vi "HandleRollerPneumatic.vi"(8 "error in (no error)":errorcluster, 10 "InitState":T1=enum."Middle", 11 "Toggle?":bool) -> (0 "error out":errorcluster, 2 "State":T1, 3 "Enqueue?":bool)   [LabVIEW 2013]
uses:
  Robot_Framework_2014/DoubleSolenoidAction.ctl
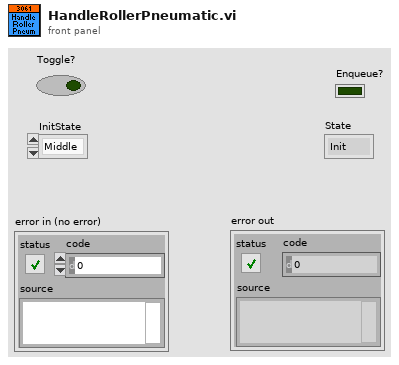
[diagram p1: front panel]
types:
  T1 = typedef "DoubleSolenoidAction.ctl" = enum16{"Init", "Middle", "In", "Out"}
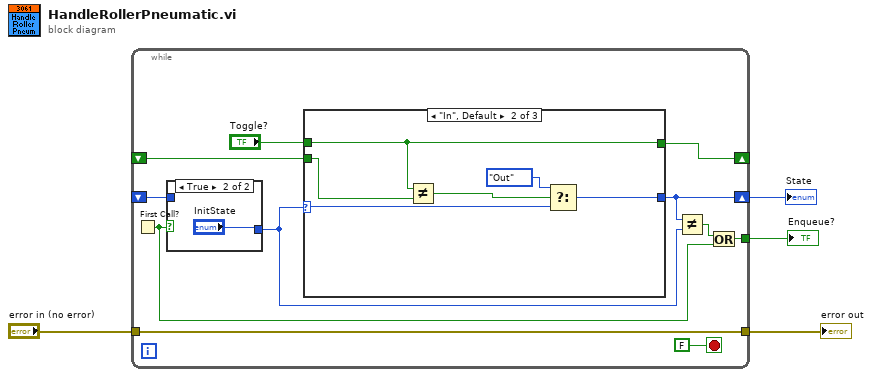
[diagram p0: block diagram]
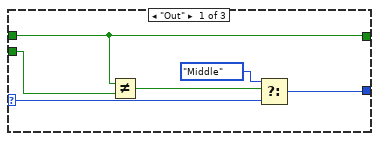
[diagram p3: hidden frame]
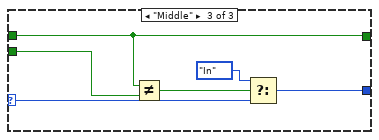
[diagram p4: hidden frame]
diagram:
  n1 = while {
    shift-right: [w9] -> w4
    shift-left: _ -> [w14]
    shift-right: [w12] -> _
    shift-left: _ -> [w11]
    tunnel: "error in (no error)" -> [w8]
    tunnel: [w8] -> w2
    tunnel: [w7] -> w1
    stop <- FALSE stop-if-true
    n2 = First Call?() -> (First Call?: T/F=w5:bool)
    n3 = case shown="True" w5 {
      tunnel: [w16 "InitState"] -> w10
      tunnel: w14 -> [w16 _]
      frame False {
      }
      frame True {
      }
    }
    n4 = case shown="\"In\", Default" w10 {
      selector: w10 -> [w21 w27 w35]
      tunnel: [w22 w28 w34] -> w9
      tunnel: [w18 w25 w32] -> w12
      tunnel: "Toggle?" -> [w18 w25 w32]
      tunnel: w11 -> [w19 w24 w31]
      frame "Out" {
        n5 = Not Equal?(x=w18, y=w19) -> (x != y?=w20:bool)
        n6 = Select(t=DoubleSolenoidAction."Middle", s=w20, f=w21) -> (s? t:f=w22:T1)
      }
      frame "In", Default {
        n7 = Not Equal?(x=w25, y=w24) -> (x != y?=w26:bool)
        n8 = Select(t=DoubleSolenoidAction."Out", s=w26, f=w27) -> (s? t:f=w28:T1)
      }
      frame "Middle" {
        n9 = Not Equal?(x=w32, y=w31) -> (x != y?=w30:bool)
        n10 = Select(t=DoubleSolenoidAction."In", s=w30, f=w35) -> (s? t:f=w34:T1)
      }
    }
    n11 = Not Equal?(x=w9, y=w10) -> (x != y?=w6:bool)
    n12 = Or(x=w6, y=w5) -> (x .or. y?=w7:bool)
  }
  "State" <- w4
  "error out" <- w2
  "Enqueue?" <- w1
